vi "ReadQuickNote.vi"(8 "error in (no error)":errorcluster, 10 "New Image":T2, 11 "GRMActor in":refnum<class "DataLoggerUI.lvclass">) -> (0 "error out":errorcluster, 2 "Image Out":T2, 3 "GRMActor out":refnum<class "DataLoggerUI.lvclass">)   [LabVIEW 2020, in "DataLogger.lvlib" / "DataLoggerUI.lvlib" / "DataLoggerUI.lvclass"]
uses:
  DataLoggerUI/DataLoggerUI.lvclass
  <vilib>/vision/Image Controls.llb/IMAQ Image.ctl
panel:
  out "Cluster":T1
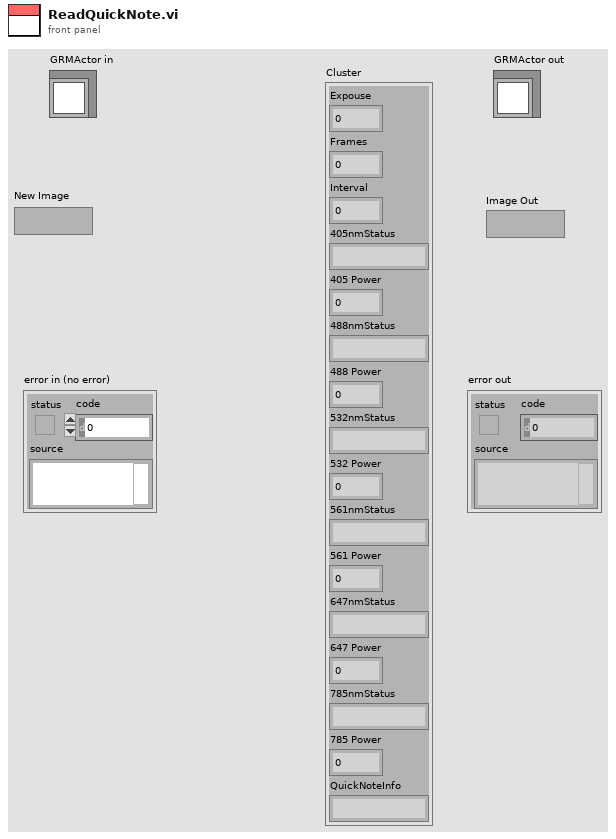
[diagram p1: front panel]
types:
  T1 = cluster{"Expouse":dbl, "Frames":dbl, "Interval":dbl, "405nmStatus":string, "405 Power":sgl, "488nmStatus":string, "488 Power":sgl, "532nmStatus":string, "532 Power":sgl, "561nmStatus":string, "561 Power":sgl, "647nmStatus":string, "647 Power":sgl, "785nmStatus":string, "785 Power":sgl, "QuickNoteInfo":string}
  T2 = typedef "IMAQ Image.ctl" = refnum<image>
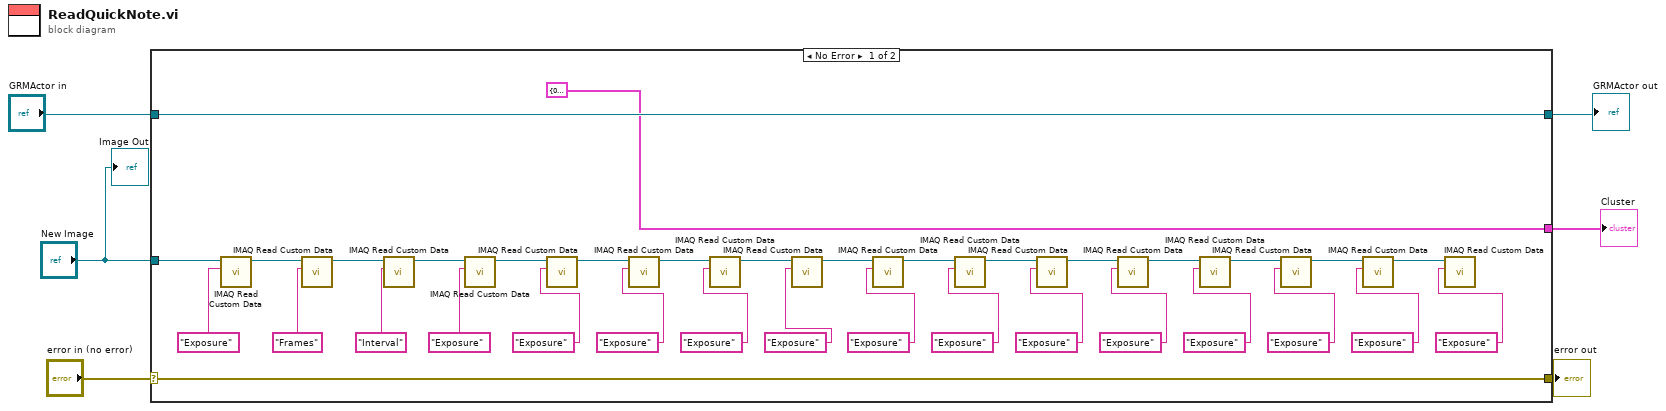
[diagram p0: block diagram]
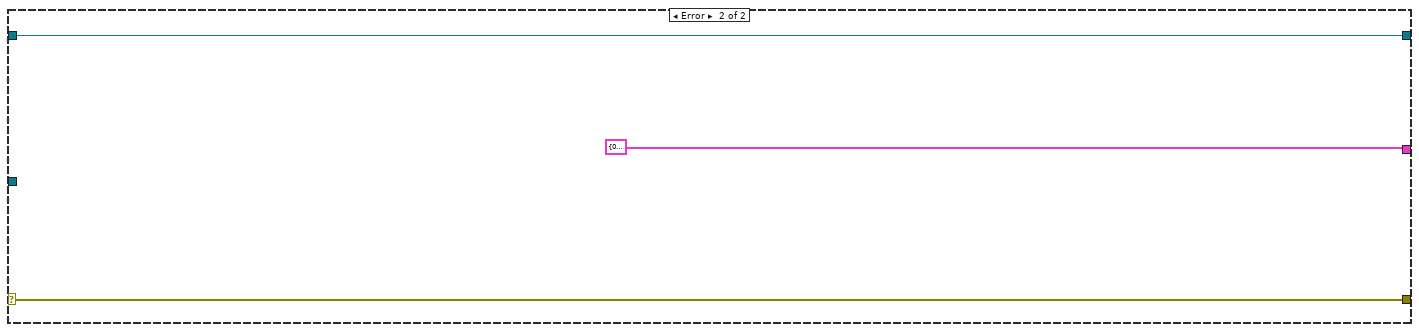
[diagram p2: hidden frame]
diagram:
  n1 = case shown="No Error" "error in (no error)" {
    selector: "error in (no error)" -> [w38 w44]
    tunnel: [w38 w44] -> w5
    tunnel: [w41 w43] -> w1
    tunnel: "GRMActor in" -> [w41 w43]
    tunnel: "New Image" -> [w39 _]
    tunnel: [T1 {"Expouse"=0.0, "Frames"=0.0, "Interval"=0.0, "405nmStatus"="", "405 Power"=0.0, "488nmStatus"="", "488 Power"=0.0, "532nmStatus"="", "532 Power"=0.0, "561nmStatus"="", "561 Power"=0.0, "647nmStatus"="", "647 Power"=0.0, "785nmStatus"="", "785 Power"=0.0, "QuickNoteInfo"=""} T1 {"Expouse"=0.0, "Frames"=0.0, "Interval"=0.0, "405nmStatus"="", "405 Power"=0.0, "488nmStatus"="", "488 Power"=0.0, "532nmStatus"="", "532 Power"=0.0, "561nmStatus"="", "561 Power"=0.0, "647nmStatus"="", "647 Power"=0.0, "785nmStatus"="", "785 Power"=0.0, "QuickNoteInfo"=""}] -> w3
    frame No Error {
      n2 = call "IMAQ Read Custom Data"("Key"="Exposure", "Image"=w39) -> ("Image (duplicate)"=w37:T2)  [unwired: 7 in, 2 out]
      n3 = call "IMAQ Read Custom Data"("Key"="Frames", "Image"=w37) -> ("Image (duplicate)"=w36:T2)  [unwired: 7 in, 2 out]
      n4 = call "IMAQ Read Custom Data"("Key"="Interval", "Image"=w36) -> ("Image (duplicate)"=w35:T2)  [unwired: 7 in, 2 out]
      n5 = call "IMAQ Read Custom Data"("Key"="Exposure", "Image"=w35) -> ("Image (duplicate)"=w34:T2)  [unwired: 7 in, 2 out]
      n6 = call "IMAQ Read Custom Data"("Key"="Exposure", "Image"=w34) -> ("Image (duplicate)"=w33:T2)  [unwired: 7 in, 2 out]
      n7 = call "IMAQ Read Custom Data"("Key"="Exposure", "Image"=w33) -> ("Image (duplicate)"=w32:T2)  [unwired: 7 in, 2 out]
      n8 = call "IMAQ Read Custom Data"("Key"="Exposure", "Image"=w32) -> ("Image (duplicate)"=w31:T2)  [unwired: 7 in, 2 out]
      n9 = call "IMAQ Read Custom Data"("Key"="Exposure", "Image"=w31) -> ("Image (duplicate)"=w30:T2)  [unwired: 7 in, 2 out]
      n10 = call "IMAQ Read Custom Data"("Key"="Exposure", "Image"=w30) -> ("Image (duplicate)"=w29:T2)  [unwired: 7 in, 2 out]
      n11 = call "IMAQ Read Custom Data"("Key"="Exposure", "Image"=w29) -> ("Image (duplicate)"=w28:T2)  [unwired: 7 in, 2 out]
      n12 = call "IMAQ Read Custom Data"("Key"="Exposure", "Image"=w28) -> ("Image (duplicate)"=w27:T2)  [unwired: 7 in, 2 out]
      n13 = call "IMAQ Read Custom Data"("Key"="Exposure", "Image"=w27) -> ("Image (duplicate)"=w26:T2)  [unwired: 7 in, 2 out]
      n14 = call "IMAQ Read Custom Data"("Key"="Exposure", "Image"=w26) -> ("Image (duplicate)"=w25:T2)  [unwired: 7 in, 2 out]
      n15 = call "IMAQ Read Custom Data"("Key"="Exposure", "Image"=w25) -> ("Image (duplicate)"=w24:T2)  [unwired: 7 in, 2 out]
      n16 = call "IMAQ Read Custom Data"("Key"="Exposure", "Image"=w24) -> ("Image (duplicate)"=w23:T2)  [unwired: 7 in, 2 out]
      n17 = call "IMAQ Read Custom Data"("Key"="Exposure", "Image"=w23) -> ()  [unwired: 7 in, 3 out]
    }
    frame Error {
    }
  }
  "error out" <- w5
  "Cluster" <- w3
  "GRMActor out" <- w1
  "Image Out" <- "New Image"
